vi "MAIN_UI Builder.vi"() -> ()   [LabVIEW 2016]
uses:
  TypeDefs/ENUM_State Main UI.ctl
  TypeDefs/ENUM_Request Main UI.ctl
  TypeDefs/Cluster_Trident Color Page.ctl
  Utility/Universal Utility/FP/FPClass/(FP)/DecFrame_FP/DecFrame_FP.lvclass
  <vilib>/Utility/error.llb/DialogType.ctl
  Utility/Universal Utility/TypeDefs_Utility/ENUM RB_Pos_Quadrant Position.ctl
  <vilib>/Utility/error.llb/Trim Whitespace.vi
panel:
  out "Copy Template":T1[](array[typedef])
  in  "Current Sequence":T1[](array[typedef])
  in  "stop":bool
  out "Version":string
  out "Action":string
  out "Next Request":T2 caption="Request"
  out "State":T3=enum."Idle"
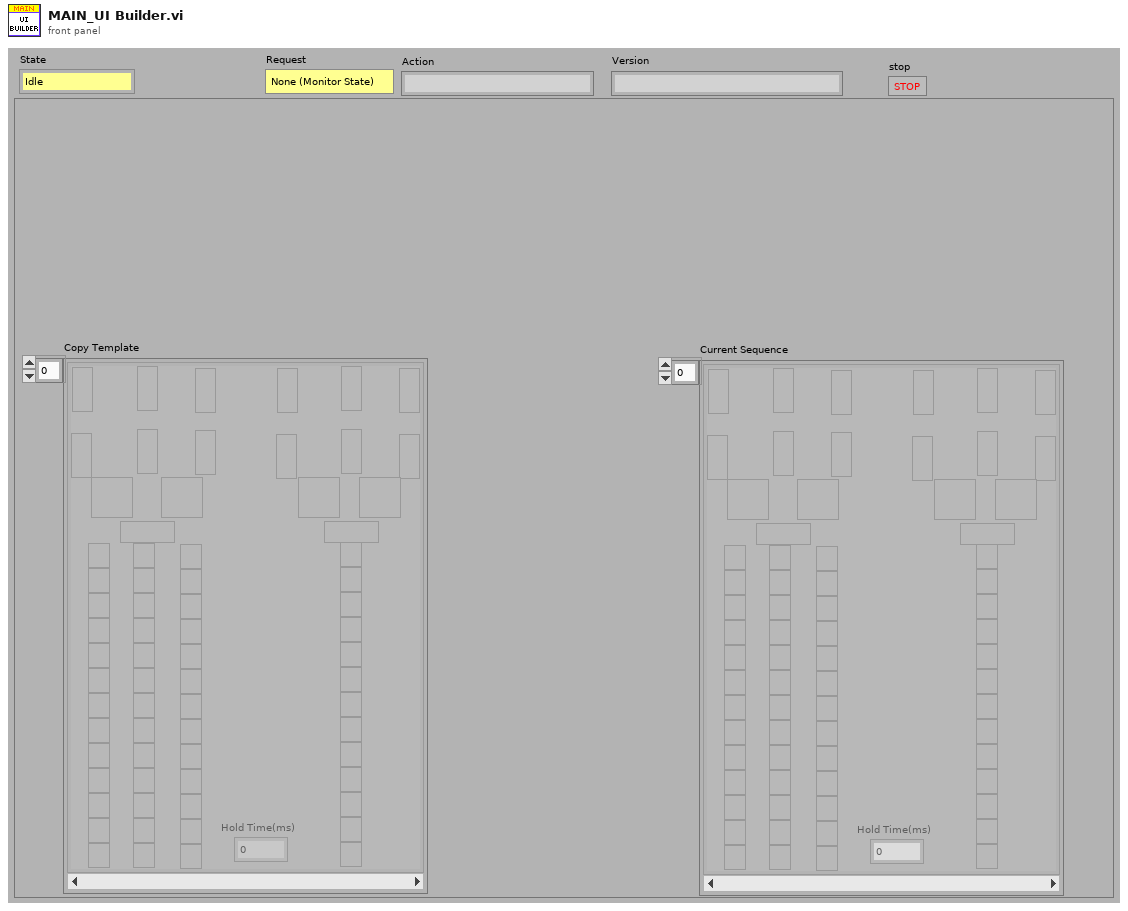
[diagram p1: front panel]
types:
  T1 = typedef "Cluster_Trident Color Page.ctl" = cluster{"0":u32, "1":u32, "2":u32, "3":u32, "4":u32, "5":u32, "6":u32, "7":u32, "8":u32, "9":u32, "10":u32, "11":u32, "12":u32, "13":u32, "14":u32, "15":u32, "16":u32, "17":u32, "18":u32, "19":u32, "20":u32, "21":u32, "22":u32, "23":u32, "24":u32, "25":u32, "26":u32, "27":u32, "28":u32, "29":u32, "30":u32, "31":u32, "32":u32, "33":u32, "34":u32, "35":u32, "36":u32, "37":u32, "38":u32, "39":u32, "40":u32, "41":u32, "42":u32, "43":u32, "44":u32, "45":u32, "46":u32, "47":u32, "48":u32, "49":u32, "50":u32, "51":u32, "52":u32, "53":u32, "54":u32, "55":u32, "56":u32, "57":u32, "58":u32, "59":u32, "60":u32, "61":u32, "62":u32, "63":u32, "64":u32, "65":u32, "66":u32, "67":u32, "68":u32, "69":u32, "Hold Time(ms)":u32}
  T2 = typedef "ENUM_Request Main UI.ctl" = enum16{"None (Monitor State)", "Request 1", "Stop Program", "SetFP Request"}
  T3 = typedef "ENUM_State Main UI.ctl" = enum16{"<Startup>", "Idle", "STATE 1", "<Shutdown>"}
  T4 = enum32{"invalid app kind", "Development System", "Run Time System", "Student Edition", "Embedded LabVIEW", "Evaluation", "Custom"}
  T5 = cluster{"App Kind":enum32{"invalid app kind", "Development System", "Run Time System", "Student Edition", "Embedded LabVIEW", "Evaluation", "Custom"}, "This VI":refnum<vi>, "Timeout":i32, "State":T3, "Request Q":refnum<queue>, "FP Data":refnum<class "DecFrame_FP.lvclass">, "Page Array":T1[]}
  T6 = typedef "ENUM RB_Pos_Quadrant Position.ctl" = enum32{"LFT-TOP", "MID-TOP", "RGT-TOP", "LFT-CTR", "MID-CTR", "RGT-CTR", "LFT-BOT", "MID-BOT", "RGT-BOT"}
  T7 = enum32{"Invalid", "Standard", "Closed", "Hidden", "Minimized", "Maximized"}
  T8 = typedef "DialogType.ctl" = u16
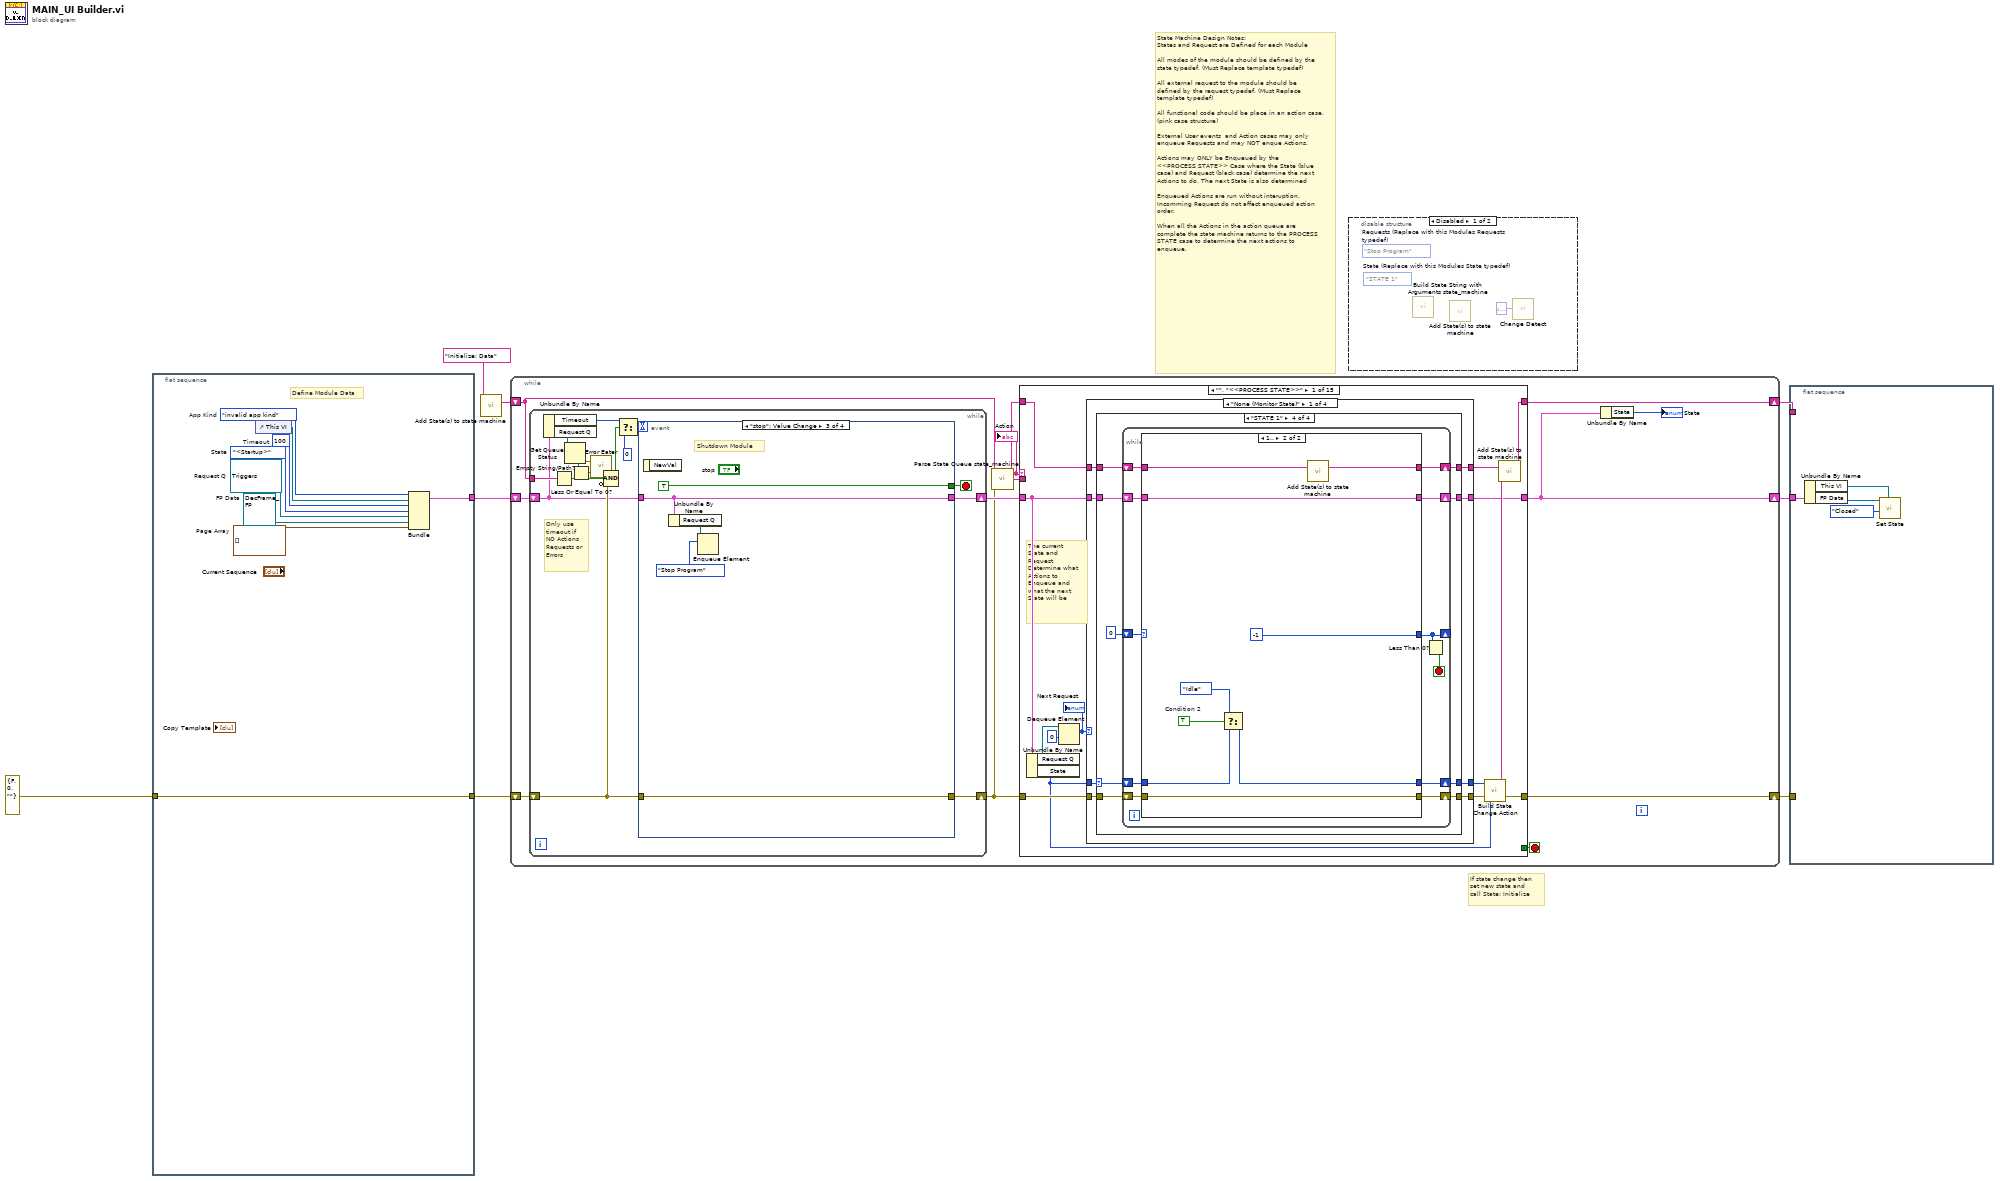
[diagram p0: block diagram]
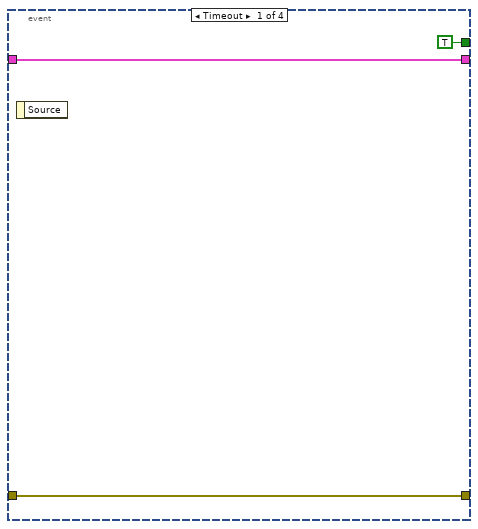
[diagram p3: hidden frame]
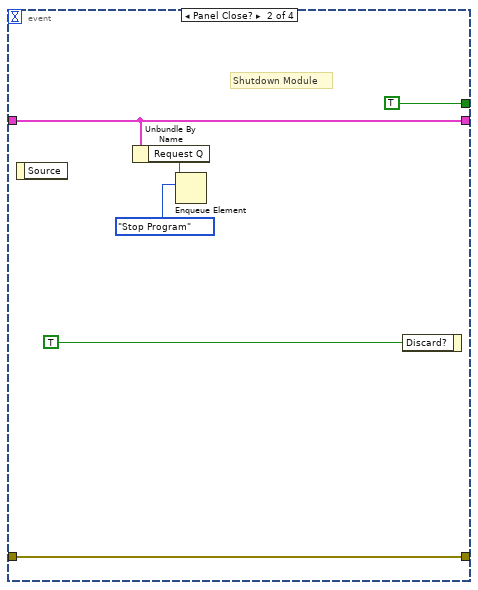
[diagram p4: hidden frame]
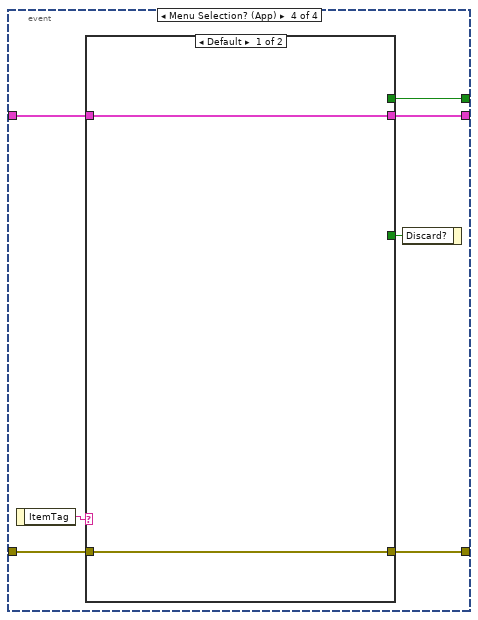
[diagram p5: hidden frame]
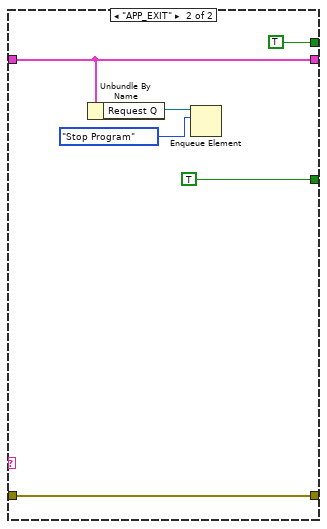
[diagram p6: hidden frame]
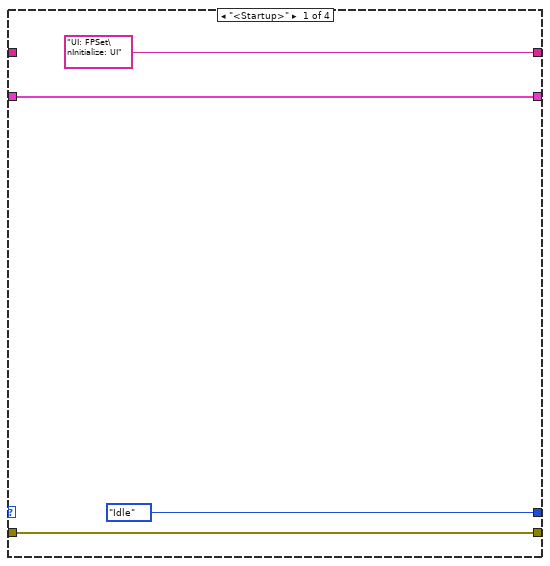
[diagram p7: hidden frame]
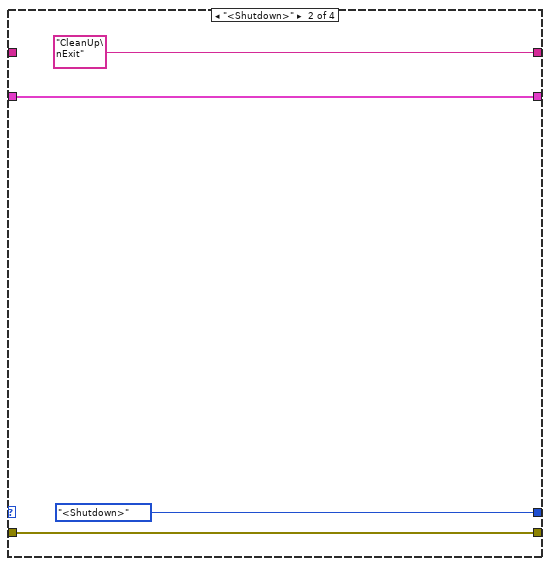
[diagram p8: hidden frame]
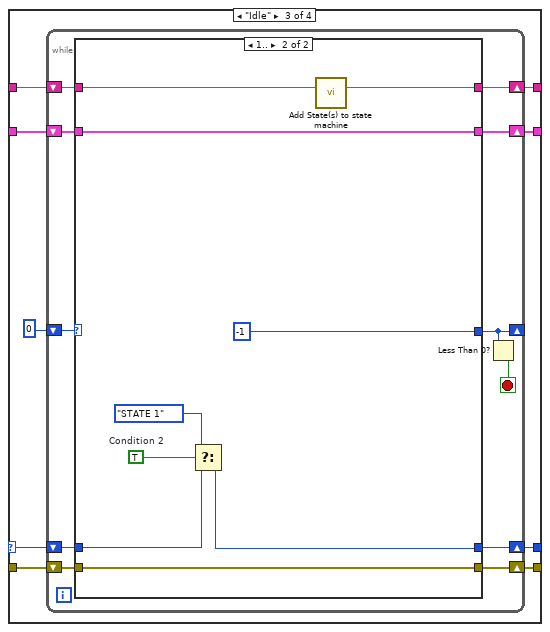
[diagram p9: hidden frame]
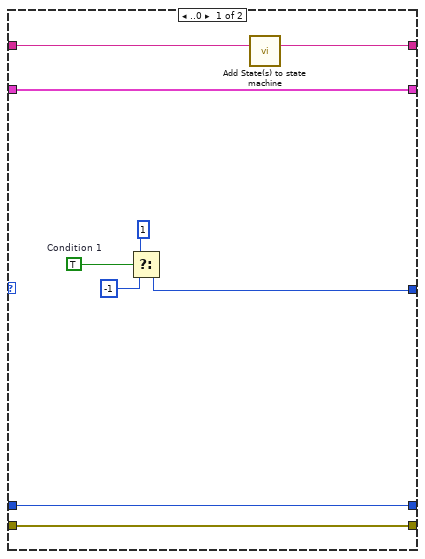
[diagram p10: hidden frame]
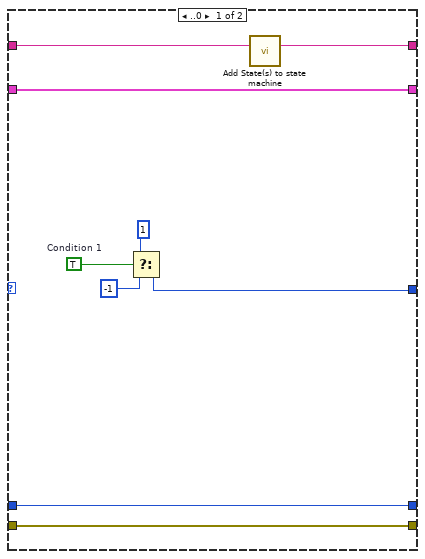
[diagram p11: hidden frame]
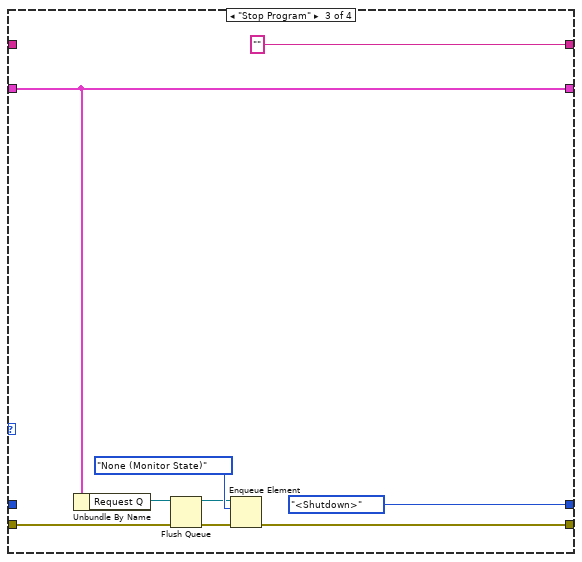
[diagram p16: hidden frame]
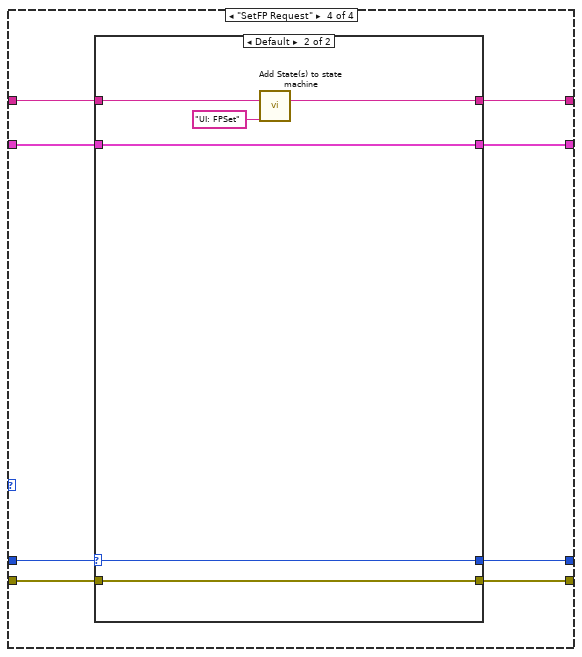
[diagram p17: hidden frame]
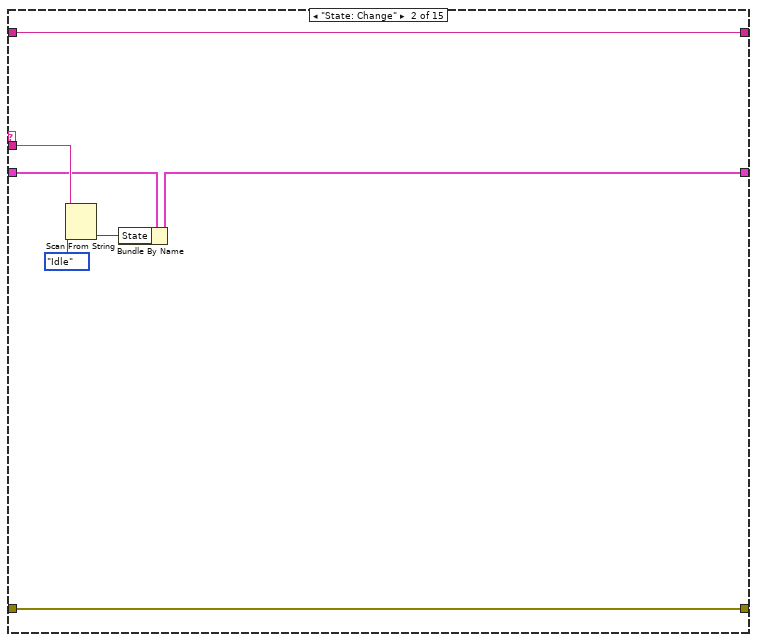
[diagram p19: hidden frame]
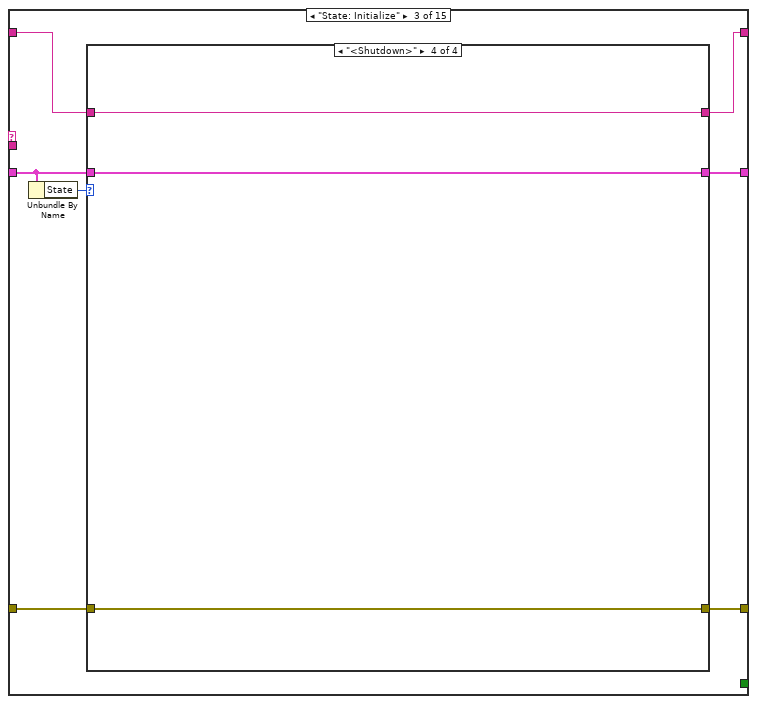
[diagram p20: hidden frame]
diagram:
  # "If state change then \nset new state and \ncall State: Initialize"
  # "State Machine Design Notes:\nStates and Request are Defined for each Module\n\nAll modes of the module should be defined by the state typedef. (Must Replace template typedef)\n\nAll external request to the module should be\ndefined by the request typedef. (Must Replace template typedef)\n\nAll functional code should be place in an action case. (pink case structure)\n\nExternal User events  and Action cases may only enqueue Requests and may NOT enque Actions.\n\nActions may ONLY be Enqueued by the\n<<PROCESS STATE>> Case where the State (blue case) and Request (black case) determine the next Actions to do. The next State is also determined\n\nEnqueued Actions are run without interuption.\nIncomming Request do not affect enqueued action order.\n\nWhen all the Actions in the action queue are complete the state machine returns to the PROCESS STATE case to determine the next actions to enqueue."
  n1 = flat-sequence {
    tunnel: errorcluster {"status"=FALSE, "code"=0, "source"=""} ("Error") -> [w17]
    tunnel: [w17] -> w6
    tunnel: [w16] -> w5
    frame #0 {
      w9 = T1[] []  # Page Array
      w10 = refnum<class "DecFrame_FP.lvclass"> refnum  # FP Data
      w12 = refnum<queue> refnum items=["None (Monitor State)", "Request 1", "Stop Program", "SetFP Request"]  # Request Q
      w11 = ENUM_State_Main_UI."<Startup>"  # State
      w14 = T4."invalid app kind"  # App Kind
      w15 = 100  # Timeout
      # "Define Module Data"
      n2 = control-ref of="This VI"() -> (w13:refnum<vi>)
      n3 = Bundle("App Kind"=w14, "This VI"=w13, "Timeout"=w15, "State"=w11, "Request Q"=w12, "FP Data"=w10, "Page Array"=w9) -> (w16:T5)  [unwired: 1 in]
    }
  }
  n4 = call "Add State(s) to state machine.vi"("State(s) in Front (\"\")"="Initialize: Data") -> ("States Out"=w8:string)  [unwired: 14 in]
  n5 = while "JKI - String-Based Queued State Machine (Basic) v1.0" {
    shift-right: [w18] -> w3
    shift-left: w5 -> [w26]
    shift-right: [w19] -> w2
    shift-left: w6 -> [w25]
    shift-right: [w28] -> w1
    shift-left: w8 -> [w21]
    stop <- w27 stop-if-true
    n6 = while {
      shift-right: [w44] -> w23
      shift-left: w25 -> [w37]
      shift-right: [w45] -> w24
      shift-left: w26 -> [w35]
      tunnel: w21 -> [w41]
      stop <- w38 stop-if-true
      # "Only use\ntimeout if\nNO Actions\nRequests or\nErrors"
      n7 = Unbundle By Name(w35) -> ("Timeout"=w39:i32, "Request Q"=w33:refnum<queue>)
      n8 = Empty String/Path?(string/path=w41) -> (empty?=w34:bool)
      n9 = Get Queue Status(queue=w33) -> (error out=w31:errorcluster, # elements in queue=w36:i32)  [unwired: 2 in, 6 out]
      n10 = Less Or Equal To 0?(x=w36) -> (x <= 0?=w32:bool)
      n11 = call "Error Eater.vi"("error in (no error)"=w31) -> ()  [unwired: 2 in]
      n12 = Compound Arithmetic op=AND(w32, w34, invert w37) -> (w43:bool)
      n13 = Select(t=w39, s=w43, f=0) -> (s? t:f=w40:i32)
      n14 = event shown="[2] \"stop\": Value Change" {
        selector: _ -> [_ _ _ _]
        dyn-events: _ -> [_ _ _ _]
        timeout: w40 -> [_ _ _ _]
        tunnel: w35 -> [w47 w52 w58 w63]
        tunnel: [w48 w54 w59 w65] -> w44
        tunnel: w37 -> [w48 w54 w59 w66]
        tunnel: [w47 w52 w58 w62] -> w45
        tunnel: [TRUE TRUE TRUE w60] -> w38
        event Timeout {
          n15 = event-data() -> ()  [unwired: 1 in, 1 out]
        }
        event Panel Close? {
          # "Shutdown Module"
          n16 = event-data() -> ()  [unwired: 1 in, 1 out]
          n17 = Unbundle By Name(w52) -> ("Request Q"=w50:refnum<queue>)
          n18 = Enqueue Element(queue=w50, element=ENUM_Request_Main_UI."Stop Program") -> ()  [unwired: 2 in, 3 out]
          n19 = event-data("Discard?"=TRUE) -> ()  [unwired: 1 in, 1 out]
        }
        event "stop": Value Change {
          # "Shutdown Module"
          n20 = event-data() -> ()  [unwired: 1 in, 1 out]
          n21 = Unbundle By Name(w58) -> ("Request Q"=w56:refnum<queue>)
          n22 = Enqueue Element(queue=w56, element=ENUM_Request_Main_UI."Stop Program") -> ()  [unwired: 2 in, 3 out]
        }
        event Menu Selection? (App) {
          n23 = event-data() -> ("ItemTag"=w64:string)  [unwired: 1 in]
          n24 = case shown="Default" w64 {
            tunnel: [w68 w74] -> w65
            tunnel: w66 -> [w68 w74]
            tunnel: [_ TRUE] -> w61
            tunnel: w63 -> [w67 w71]
            tunnel: [w67 w71] -> w62
            tunnel: [_ TRUE] -> w60
            frame Default {
            }
            frame "APP_EXIT" {
              n25 = Unbundle By Name(w71) -> ("Request Q"=w70:refnum<queue>)
              n26 = Enqueue Element(queue=w70, element=ENUM_Request_Main_UI."Stop Program") -> ()  [unwired: 2 in, 3 out]
            }
          }
          n27 = event-data("Discard?"=w61) -> ()  [unwired: 1 in, 1 out]
        }
      }
    }
    n28 = call "Parse State Queue state_machine.vi"("State Queue"=w21, "Error In (no error)"=w23) -> ("Remaining States"=w30:string, "Current State"=w20:string, "Arguments"=w29:string)  [unwired: 11 in]
    "Action" <- w20
    n29 = case shown="\"\", \"<<PROCESS STATE>>\"" w20 {
      selector: w20 -> [_ _ _ w259 _ _ _ _ _ _ _ _ _ _ _]
      tunnel: w30 -> [w78 w237 w240 w258 w268 w287 w289 w293 w307 w310 w313 w324 w325 w329 w332]
      tunnel: w29 -> [_ w236 _ _ _ _ _ _ _ _ _ _ _ _ _]
      tunnel: w24 -> [w79 w235 w244 w261 w271 w282 w292 w294 w304 w312 w314 w319 w326 w328 w331]
      tunnel: [w80 w238 w241 w263 w269 w286 w291 w295 w296 w311 w315 w320 w327 w330 w333] -> w19
      tunnel: w23 -> [w83 w238 w242 w262 w272 w286 w291 w295 w296 w311 w315 w321 w327 w330 w333]
      tunnel: [w87 w237 w239 w258 w268 w287 w289 w293 w307 w310 w313 w324 w325 w329 w332] -> w28
      tunnel: [_ _ _ _ _ _ TRUE _ _ _ _ _ _ _ _] -> w27
      tunnel: [w76 w234 w243 w261 w270 w282 w292 w294 w308 w312 w314 w318 w326 w328 w331] -> w18
      frame "", "<<PROCESS STATE>>" {
        # "The current\nState and \nRequest\nDetermine what\nActions to\nEnqueue and\nwhat the next\nState will be"
        n30 = Unbundle By Name(w79) -> ("Request Q"=w85:refnum<queue>, "State"=w82:T3)
        n31 = Dequeue Element(queue=w85, timeout in ms (-1)=0) -> (element=w75:T2)  [unwired: 1 in, 3 out]
        "Next Request" <- w75
        n32 = case shown="\"None (Monitor State)\"" w75 {
          selector: w75 -> [_ w181 _ _]
          tunnel: w78 -> [w92 w188 _ w218]
          tunnel: [w89 w187 w212 w217] -> w76
          tunnel: [w93 w186 w205 w214] -> w80
          tunnel: w83 -> [w94 w185 w206 w215]
          tunnel: w82 -> [w95 w184 _ w220]
          tunnel: [w88 w183 ENUM_State_Main_UI."<Shutdown>" ("State") w216] -> w81
          tunnel: w79 -> [w90 w182 w212 w219]
          tunnel: [w91 w180 "" ("Remaining States") w221] -> w77
          frame "None (Monitor State)" {
            n33 = case shown="\"STATE 1\"" w95 {
              selector: w95 -> [_ _ w110 w148]
              tunnel: w94 -> [w99 w103 w109 w147]
              tunnel: [w99 w103 w105 w143] -> w93
              tunnel: w92 -> [_ _ w112 w150]
              tunnel: ["UI: FPSet\nInitialize: UI" "CleanUp\nExit" w107 w145] -> w91
              tunnel: w90 -> [w98 w102 w111 w149]
              tunnel: [w98 w102 w106 w144] -> w89
              tunnel: [ENUM_State_Main_UI."Idle" ("State") ENUM_State_Main_UI."<Shutdown>" ("State") w104 w142] -> w88
              frame "<Startup>" {
              }
              frame "<Shutdown>" {
              }
              frame "Idle" {
                n34 = while {
                  shift-right: [w115] -> w105
                  shift-left: w109 -> [w116]
                  shift-right: [w117] -> w104
                  shift-left: w110 -> [w118]
                  shift-right: [w113] -> w106
                  shift-left: w111 -> [w114]
                  shift-right: [w121] -> w107
                  shift-left: w112 -> [w122]
                  shift-right: [w119] -> _
                  shift-left: 0 -> [w123]
                  stop <- w120 stop-if-true
                  n35 = case shown="1.." w123 {
                    tunnel: w122 -> [w132 w141]
                    tunnel: [w131 w140] -> w121
                    tunnel: [w126 -1 ("t")] -> w119
                    tunnel: w118 -> [w124 w135]
                    tunnel: [w124 w134] -> w117
                    tunnel: w116 -> [w130 w139]
                    tunnel: [w130 w139] -> w115
                    tunnel: w114 -> [w129 w138]
                    tunnel: [w129 w138] -> w113
                    frame ..0 {
                      w125 = TRUE  # Condition 1
                      n36 = Select(t=1, s=w125, f=-1) -> (s? t:f=w126:i32)
                      n37 = call "Add State(s) to state machine.vi"("State(s) in (\"\")"=w132) -> ("States Out"=w131:string)  [unwired: 14 in]
                    }
                    frame 1.. {
                      w137 = TRUE  # Condition 2
                      n38 = Select(t=ENUM_State_Main_UI."STATE 1", s=w137, f=w135) -> (s? t:f=w134:T3)
                      n39 = call "Add State(s) to state machine.vi"("State(s) in (\"\")"=w141) -> ("States Out"=w140:string)  [unwired: 14 in]
                    }
                  }
                  n40 = Less Than 0?(x=w119) -> (x < 0?=w120:bool)
                }
              }
              frame "STATE 1" {
                n41 = while {
                  shift-right: [w153] -> w143
                  shift-left: w147 -> [w154]
                  shift-right: [w155] -> w142
                  shift-left: w148 -> [w156]
                  shift-right: [w151] -> w144
                  shift-left: w149 -> [w152]
                  shift-right: [w159] -> w145
                  shift-left: w150 -> [w160]
                  shift-right: [w157] -> _
                  shift-left: 0 -> [w161]
                  stop <- w158 stop-if-true
                  n42 = case shown="1.." w161 {
                    tunnel: w160 -> [w170 w179]
                    tunnel: [w169 w178] -> w159
                    tunnel: [w164 -1 ("t")] -> w157
                    tunnel: w156 -> [w162 w173]
                    tunnel: [w162 w172] -> w155
                    tunnel: w154 -> [w168 w177]
                    tunnel: [w168 w177] -> w153
                    tunnel: w152 -> [w167 w176]
                    tunnel: [w167 w176] -> w151
                    frame ..0 {
                      w163 = TRUE  # Condition 1
                      n43 = Select(t=1, s=w163, f=-1) -> (s? t:f=w164:i32)
                      n44 = call "Add State(s) to state machine.vi"("State(s) in (\"\")"=w170) -> ("States Out"=w169:string)  [unwired: 14 in]
                    }
                    frame 1.. {
                      w175 = TRUE  # Condition 2
                      n45 = Select(t=ENUM_State_Main_UI."Idle", s=w175, f=w173) -> (s? t:f=w172:T3)
                      n46 = call "Add State(s) to state machine.vi"("State(s) in (\"\")"=w179) -> ("States Out"=w178:string)  [unwired: 14 in]
                    }
                  }
                  n47 = Less Than 0?(x=w157) -> (x < 0?=w158:bool)
                }
              }
            }
          }
          frame "Request 1" {
            n48 = case shown="\"Idle\"" w184 {
              selector: w184 -> [w190 w193 w197 w201]
              tunnel: w188 -> [w192 w196 w199 w203]
              tunnel: w182 -> [w191 w195 w200 w204]
              tunnel: [w191 w195 w200 w204] -> w187
              tunnel: [w192 w196 w199 w203] -> w180
              tunnel: [w189 w194 w198 w202] -> w186
              tunnel: w185 -> [w189 w194 w198 w202]
              tunnel: w181 -> [_ _ _ _]
              tunnel: [w190 w193 w197 w201] -> w183
              frame "Idle" {
              }
              frame "STATE 1" {
              }
              frame "<Shutdown>" {
              }
              frame "<Startup>" {
              }
            }
          }
          frame "Stop Program" {
            n49 = Unbundle By Name(w212) -> ("Request Q"=w209:refnum<queue>)
            n50 = Flush Queue(queue=w209, error in (no error)=w206) -> (queue out=w208:refnum<queue>, error out=w207:errorcluster)  [unwired: 1 out]
            n51 = Enqueue Element(queue=w208, element=ENUM_Request_Main_UI."None (Monitor State)", error in (no error)=w207) -> (error out=w205:errorcluster)  [unwired: 1 in, 2 out]
          }
          frame "SetFP Request" {
            n52 = case shown="Default" w220 {
              selector: w220 -> [w222 w227]
              tunnel: [w224 w230] -> w221
              tunnel: w219 -> [w223 w228]
              tunnel: w218 -> [w224 w231]
              tunnel: [w223 w228] -> w217
              tunnel: [w222 w227] -> w216
              tunnel: w215 -> [w225 w226]
              tunnel: [w225 w226] -> w214
              frame "<Shutdown>" {
              }
              frame Default {
                n53 = call "Add State(s) to state machine.vi"("State(s) in (\"\")"=w231, "State(s) at Back (\"\")"="UI: FPSet") -> ("States Out"=w230:string)  [unwired: 13 in]
              }
            }
          }
        }
        n54 = call "Build State Change Action.vi"("Current State"=w82, "Target State"=w81) -> ("Action String Out"=w86:string)  [unwired: 3 in]
        n55 = call "Add State(s) to state machine.vi"("State(s) in (\"\")"=w77, "State(s) at Back (\"\")"=w86) -> ("States Out"=w87:string)  [unwired: 13 in]
      }
      frame "State: Change" {
        n56 = Scan From String(input string=w236, default 1=ENUM_State_Main_UI."Idle" ("State")) -> (output 1=w232:T3)  [unwired: 3 in, 3 out]
        n57 = Bundle By Name(cluster=w235, "State"=w232) -> (w234:T5)
      }
      frame "State: Initialize" {
        n58 = Unbundle By Name(w244) -> ("State"=w245:T3)
        n59 = case shown="\"<Shutdown>\"" w245 {
          tunnel: w244 -> [w248 w251 w254 w257]
          tunnel: [w248 w251 w254 w257] -> w243
          tunnel: w242 -> [w247 w250 w253 w256]
          tunnel: [w247 w250 w253 w256] -> w241
          tunnel: w240 -> [w246 w249 w252 w255]
          tunnel: [w246 w249 w252 w255] -> w239
          frame "Idle" {
          }
          frame "<Startup>" {
          }
          frame "STATE 1" {
          }
          frame "<Shutdown>" {
          }
        }
      }
      frame Default {
        w266 = 42 items=["No error", "Argument error", "Memory is full", "Out of zone", "End of file", "File already open", "Generic file I/O error", "File not found", "File permission error", "Disk is full", "Duplicate path", "Too many files open", "System feature not enabled", "Resource file not found", "Cannot add resource", "Resource not found", "Image not found", "Image memory error", "Pen does not exist", "Config type invalid", "Config token not found", "Config parse error", "Config memory error", "Bad external code format", "Bad external code offset", "External code not present", "Null window", "Destroy window error", "Null menu", "Print aborted", "Bad print record", "Print driver error", "Windows error during printing", "Memory error during printing", "Print dialog error", "Generic print error", "Invalid device refnum", "Device not found", "Device parameter error", "Device unit error", "Cannot open device", "Device call aborted", "Generic error", "Cancelled by user", "Object ID too low", "Object ID too high", "Object not in heap", "Unknown heap", "Unknown object (invalid DefProc)", "Unknown object (DefProc not in table)", "Message out of range", "Invalid (null) method", "Unknown message", "Manager call not supported", "Bad address", "Network operation in progress", "Network operation timed out", "Connection is busy", "Network attribute not supported", "Network error", "Address in use", "System out of memory", "Connection aborted", "Connection refused", "Not connected", "Already connected", "Connection closed", "Initialization error (interapplication manager)", "Bad occurrence", "Wait on unbound occurrence handler", "Occurrence queue overflow", "Datalog type conflict", "Unused", "Unrecognized type (interapplication manager)", "Memory corrupt", "Failed to make temporary DLL", "Old CIN version", "Drag socket not found", "Failed to load drop-object", "Failed to register OLE object", "Failed to release OLE object", "Format specifier type mismatch", "Unknown format specifier", "Too few format specifiers", "Too many format specifiers", "Scan failed", "Newer CIN version", "Error converting to variant", "Runtime menu error", "Password tampered", "Variant attribute not found", "Incompatible variant data type", "Event data is not available", "Event Store is not present", "Occurrence is not found", "Event Queue is not created", "Event info is not available", "Refnum passed is NULL", "Error retrieving Class GUID", "Error retrieving CoClass GUID", "Error retrieving TypeLib GUID.", "Bad built application magic bytes.", "Specific driver is different from the specific driver associated with the Logical Name.", "There is no session opened to the class driver.", "Max Error", "MAX - Error with config objects", "MAX - Error loading configuration", "MAX - Group not supported"]
        n60 = Format Into String(format string="Unable to process Action\nNo Action Case is defined for\n%s" ("message"), error in=w262, w259) -> (resulting string=w265:string, error out=w264:errorcluster)  [unwired: 1 in]
        n61 = call <vilib>:"Error Cluster From Error Code.vi"("show call chain? (False)"=TRUE, "error in (no error)"=w264, "error message (\"\")"=w265, "error code (0)"=w266) -> ("error out"=w263:errorcluster)  [unwired: 5 in]
      }
      frame "Error Handler" {
        n62 = case shown="False" FALSE {
          tunnel: w272 -> [w278 _]
          tunnel: [w277 w280] -> w270
          tunnel: w271 -> [w277 w280]
          tunnel: [errorcluster {"status"=FALSE, "code"=0, "source"=""} ("error out") errorcluster {"status"=FALSE, "code"=0, "source"=""} ("error out")] -> w269
          frame False {
            w274 = T8 2 items=["no dialog", "OK message", "continue or stop message", "OK message + warnings", "continue/stop + warnings"] ("type of dialog (OK msg:1)")
            # "Display error"
            n63 = call <vilib>:"General Error Handler.vi"("type of dialog (OK msg:1)"=w274, "error in (no error)"=w278) -> ("error out"=w275:errorcluster)  [unwired: 9 in, 4 out]
            n64 = flat-sequence {
              tunnel: w275 -> [_]
              frame #0 {
                n65 = Wait (ms)(milliseconds to wait=u32 2000) -> ()  [unwired: 1 out]
              }
            }
          }
          frame True {
            # "Clear error"
          }
        }
      }
      frame "CleanUp" {
        # "Destroy and open refs"
        n66 = Unbundle By Name(w282) -> ("This VI"=w288:refnum<vi>, "Request Q"=w284:refnum<queue>)
        n67 = Close Reference(reference=w288) -> (error out=w285:errorcluster)  [unwired: 1 in]
        n68 = Release Queue(queue=w284) -> (error out=w283:errorcluster)  [unwired: 2 in, 2 out]
        n69 = call <vilib>:"Clear Errors.vi"("error in (no error)"=w285) -> ()  [unwired: 5 in, 2 out]
        n70 = call <vilib>:"Clear Errors.vi"("error in (no error)"=w283) -> ()  [unwired: 5 in, 2 out]
      }
      frame "Exit" {
      }
      frame "---------- Initialize ----------" {
      }
      frame "Initialize: Data" {
        w297 = i16 -2  # Border Spacing
        w301 = 0  # Decoration Index
        w302 = u16 0  # Monitor #
        # "INI Data"
        n71 = Unbundle By Name(w304) -> ("FP Data"=w303:refnum<class "DecFrame_FP.lvclass">)
        n72 = call-dynamic "Setup DecFrame Data.vi"("Border Spacing"=w297, "Monitor #"=w302, "FPLocation"=ENUM_RB_Pos_Quadrant_Position."LFT-TOP", "Decoration Index"=w301, "(FP)"=w303) -> ("(FP) Out"=w299:refnum<class "DecFrame_FP.lvclass">)  [unwired: 5 in, 1 out]
        n73 = property class="App"() -> ("App.Kind"=w300:T4)  [unwired: 2 in, 2 out]
        n74 = Obtain Queue(element data type=ENUM_Request_Main_UI."Request 1" ("Triggers")) -> (queue out=w306:refnum<queue>)  [unwired: 4 in, 2 out]
        n75 = Bundle By Name(cluster=w304, "FP Data"=w299, "App Kind"=w300, "Request Q"=w306) -> (w308:T5)
      }
      frame "Initialize: UI" {
        # "Setup UI indicators and controls"
        n76 = call "[Version] - Get Application Main.vi"() -> ("Version"=→"Version":string)
      }
      frame "---------- UI ----------" {
      }
      frame "UI: FPSet" {
        # "Set FP"
        n77 = Unbundle By Name(w319) -> ("This VI"=w323:refnum<vi>, "FP Data"=w322:refnum<class "DecFrame_FP.lvclass">)
        n78 = call-dynamic "Set State.vi"("VI Ref"=w323, "Error"=w321, "State"=T7."Standard", "(FP)"=w322) -> ("Error Out"=w320:errorcluster, "(FP) Out"=w317:refnum<class "DecFrame_FP.lvclass">)  [unwired: 5 in, 1 out]
        n79 = Bundle By Name(cluster=w319, "FP Data"=w317) -> (w318:T5)
      }
      frame "---------- Action ----------" {
      }
      frame "Action: One" {
      }
      frame "Action: Two" {
      }
    }
    n80 = Unbundle By Name(w18) -> ("State"=→"State":T3)
  }
  n81 = disable-structure shown="Disabled" {
    frame Disabled {
      (unwired) ENUM_Request_Main_UI."Stop Program"  # Requests (Replace with this Modules Requests typedef)
      (unwired) ENUM_State_Main_UI."STATE 1"  # State (Replace with this Modules State typedef)
      n82 = call "Build State String with Arguments state_machine.vi"() -> ()  [unwired: 6 in, 1 out]
      n83 = call "Add State(s) to state machine.vi"() -> ()  [unwired: 15 in, 1 out]
      n84 = call "Change Detect.vi"("Value"=variant) -> ()  [unwired: 4 in, 1 out]
    }
    frame Enabled {
    }
  }
  n85 = flat-sequence {
    tunnel: w3 -> [w338]
    tunnel: w2 -> [_]
    tunnel: w1 -> [_]
    frame #0 {
      n86 = Unbundle By Name(w338) -> ("This VI"=w336:refnum<vi>, "FP Data"=w337:refnum<class "DecFrame_FP.lvclass">)
      n87 = call-dynamic "Set State.vi"("VI Ref"=w336, "State"=T7."Closed", "(FP)"=w337) -> ()  [unwired: 6 in, 3 out]
    }
  }
